vi "FastLocalizeCPU.vi"(5 "Image":T1, 7 "debug image":T1) -> (0 "median":sgl, 1 "xcorpos":cluster{"XCor X":sgl, "XCor Y":sgl}, 2 "debug image":T1(plugin-control), 3 "COM":cluster{"comX":sgl, "comY":sgl})   [LabVIEW 2011]
uses:
  <vilib>/vision/Image Controls.llb/IMAQ Image.ctl
  cudatrack-debug.dll
panel:
  in  "XCor X":sgl
  in  "XCor Y":sgl
  in  "comX":sgl
  in  "comY":sgl
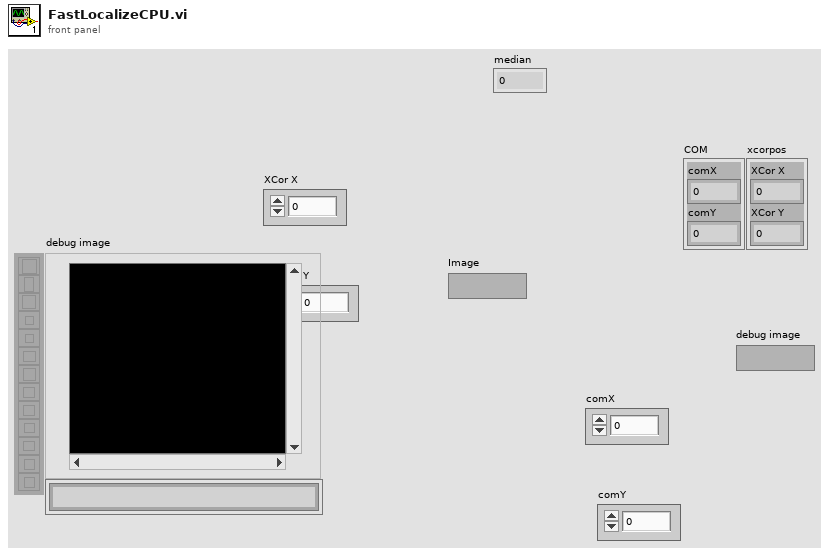
[diagram p1: front panel]
types:
  T1 = typedef "IMAQ Image.ctl" = refnum<image>
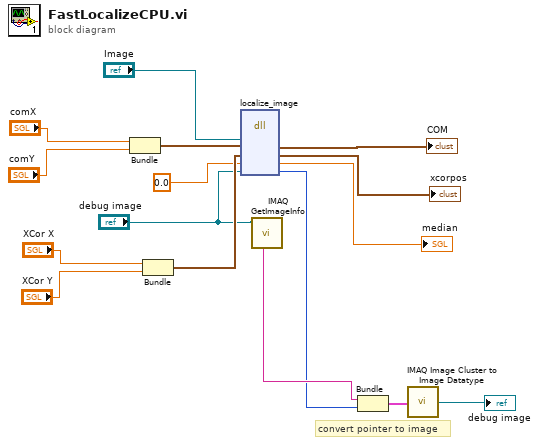
[diagram p0: block diagram]
diagram:
  # "convert pointer to image"
  n1 = Bundle("comX"="comX", "comY"="comY") -> (w14:cluster{"comX":sgl, "comY":sgl})  [unwired: 1 in]
  n2 = Bundle("XCor X"="XCor X", "XCor Y"="XCor Y") -> (w11:cluster{"XCor X":sgl, "XCor Y":sgl})  [unwired: 1 in]
  n3 = dll-call lib="D:/jcnossen1/cudaqi-tracker/cudatrack/cudatrack-debug.dll" fn="localize_image"("image"="Image", "COM"=w14, "xcorpos"=w11, "median"=sgl 0.0, "debugImage"="debug image") -> ("COM"=→"COM":cluster{"comX":sgl, "comY":sgl}, "xcorpos"=→"xcorpos":cluster{"XCor X":sgl, "XCor Y":sgl}, "median"=→"median":sgl, "debugImage"=w1:u64)  [unwired: 5 in, 2 out]
  n4 = call "IMAQ GetImageInfo"("Image"="debug image") -> ("Image Name"=w3:string)  [unwired: 3 in, 7 out]
  n5 = Bundle("Image Name"=w3, "debugImage"=w1) -> (w4:cluster{"Image Name":string, "debugImage":u64})  [unwired: 1 in]
  n6 = call <vilib>:"IMAQ Image Cluster to Image Datatype.vi"("Image"=w4) -> ("Image (dup)"=→"debug image":T1)
